vi "BRig_Host_dataRunState__entryAdd_v2.vi"(0 "input_dataPlot":u16[][](array[numeric]), 1 "input_dataTS":u16[][](array[numeric]), 2 "input_idx":i32[](array[numeric]), 4 "input_nTrial":u16, 5 "input_LorR":u16, 7 "input_sSelection":u16, 9 "input_tSelection":u16, 11 "input_tSelectionPlot":u16, 13 "input_iSelection":u16) -> (14 "output_dataPlot":u16[][](array[numeric]), 15 "output_dataTS":u16[][](array[numeric]), 16 "output_idx":i32[](array[numeric]), 18 "output_updatePlot":bool)   [LabVIEW 2014]
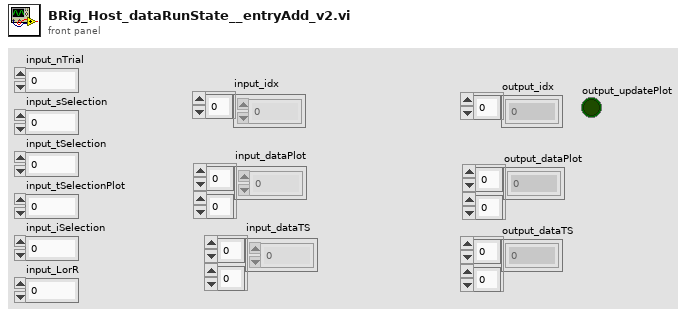
[diagram p1: front panel]
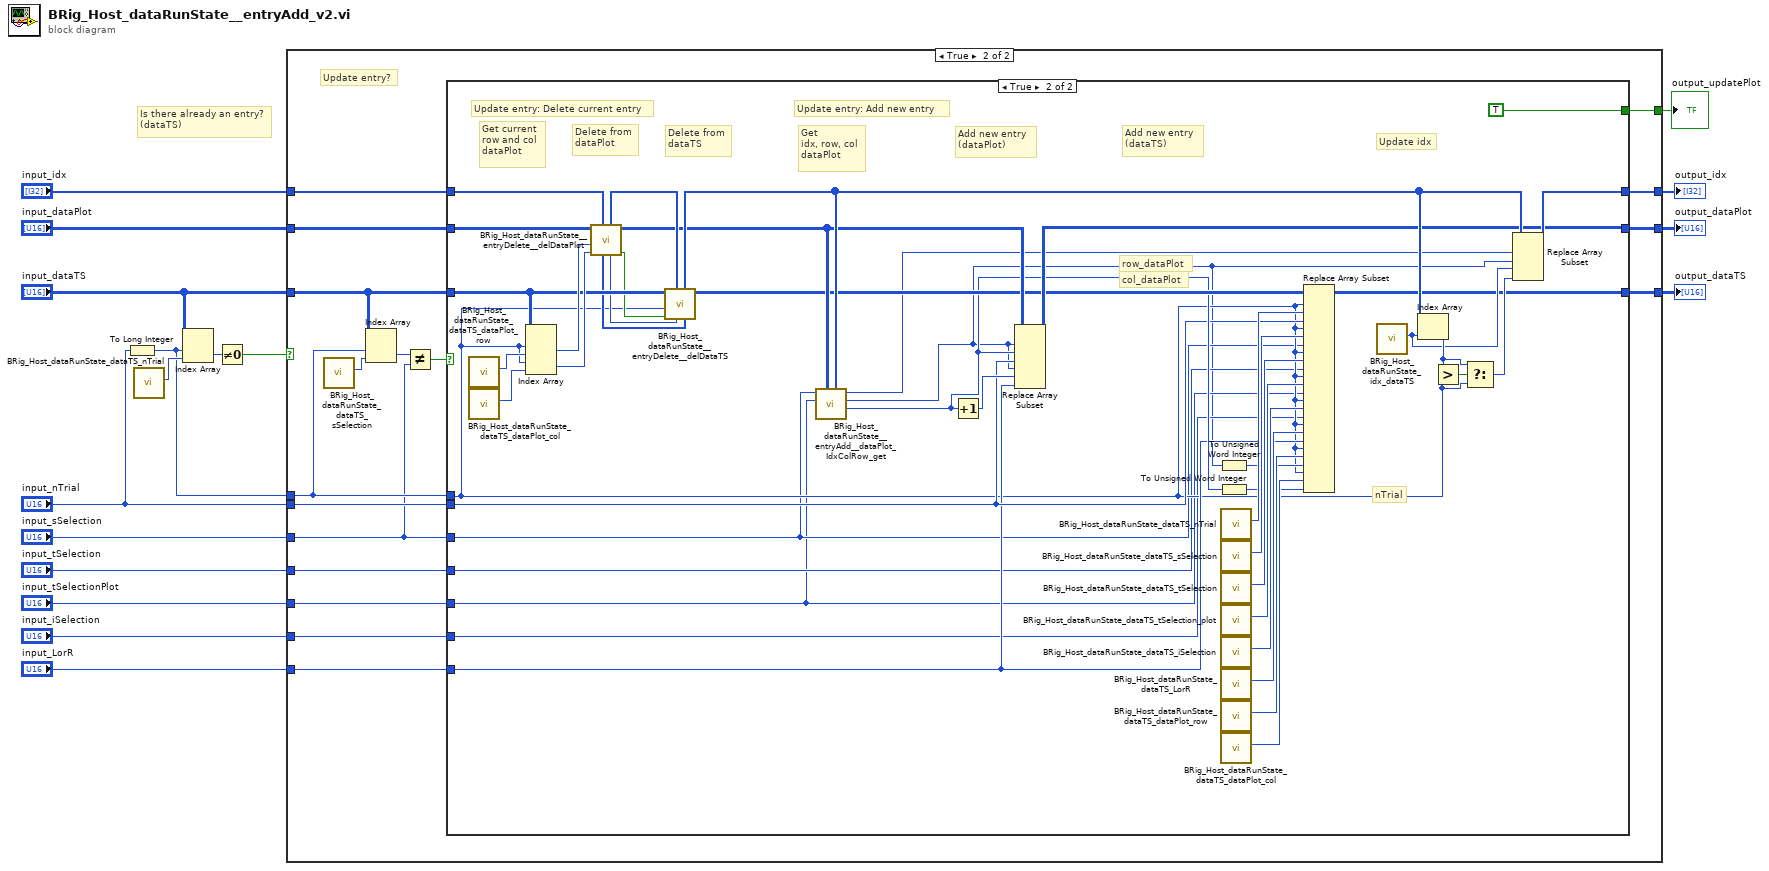
[diagram p0: block diagram]
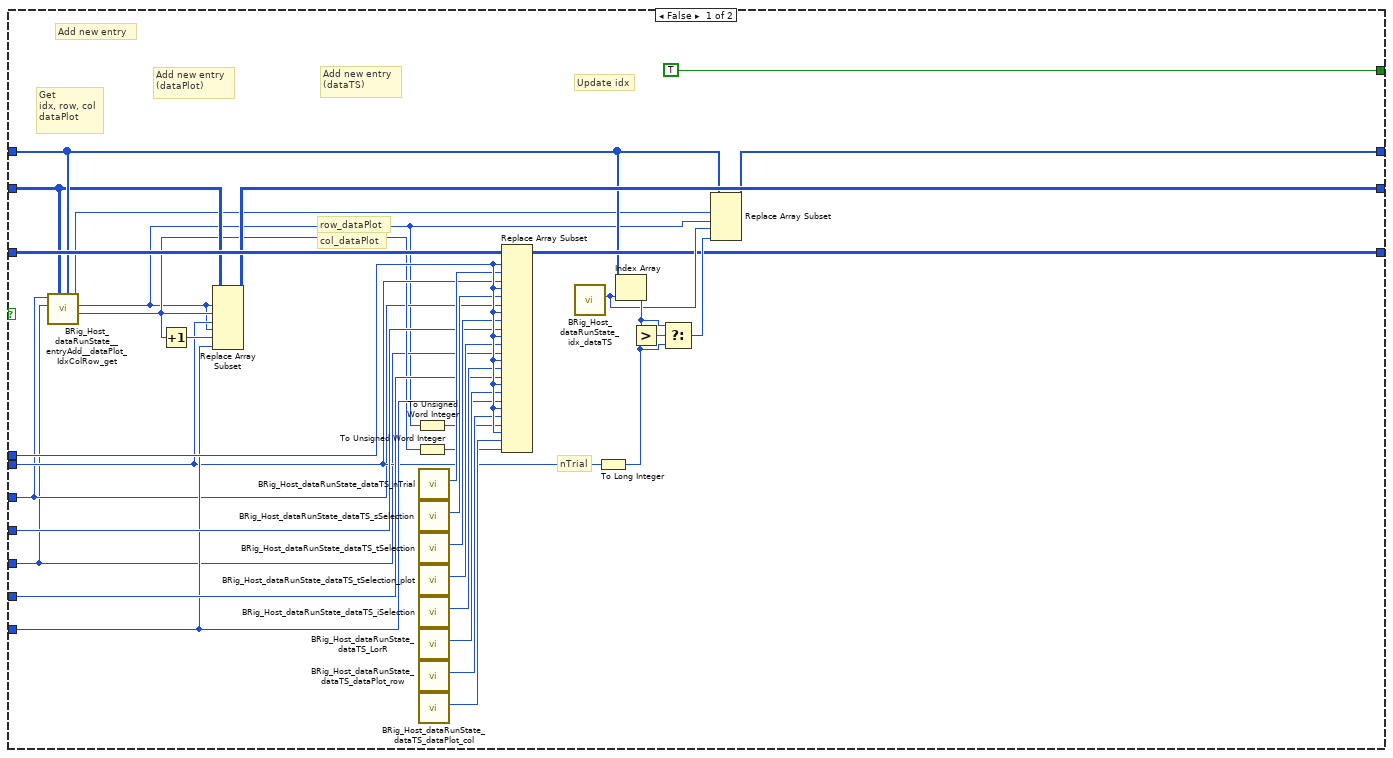
[diagram p2: hidden frame]
diagram:
  # "Is there already an entry?\n(dataTS)"
  n1 = To Long Integer(number="input_nTrial") -> (32bit integer=w13:i32)
  n2 = call "BRig_Host_dataRunState_dataTS_nTrial.vi"() -> ("output_idx_dataTS_nTrial"=w17:i32)  [unwired: 11 in]
  n3 = Index Array(array="input_dataTS", index (row)=w13, index (col)=w17) -> (element=w16:u16)
  n4 = Not Equal To 0?(x=w16) -> (x != 0?=w15:bool)
  n5 = case shown="True" w15 {
    tunnel: "input_nTrial" -> [w27 w57]
    tunnel: w13 -> [w49 w59]
    tunnel: "input_dataTS" -> [w50 w61]
    tunnel: "input_idx" -> [w24 w65]
    tunnel: "input_dataPlot" -> [w23 w63]
    tunnel: "input_sSelection" -> [w20 w51]
    tunnel: "input_tSelectionPlot" -> [w19 w58]
    tunnel: "input_iSelection" -> [w36 w54]
    tunnel: "input_LorR" -> [w35 w56]
    tunnel: [w38 w64] -> w4
    tunnel: [w39 w62] -> w3
    tunnel: [w30 w60] -> w2
    tunnel: "input_tSelection" -> [w37 w55]
    tunnel: [TRUE w53] -> w1
    frame False {
      # "Get\nidx, row, col\ndataPlot"
      # "nTrial"
      # "row_dataPlot"
      # "col_dataPlot"
      # "Update idx"
      # "Add new entry\n(dataPlot)"
      # "Add new entry"
      # "Add new entry\n(dataTS)"
      n6 = call "BRig_Host_dataRunState__entryAdd__dataPlot_IdxColRow_get.vi"("input_idx"=w24, "input_dataPlot"=w23, "input_tSelectionPlot"=w19, "input_sSelection"=w20) -> ("output_col_dataPlot"=w21:i32, "output_row_dataPlot"=w18:i32, "output_idx_dataPlot"=w22:i32)  [unwired: 5 in]
      n7 = Increment(x=w21) -> (x+1=w40:i32)
      n8 = Replace Array Subset(array=w23, new element #1=w27, index (row) #1=w18, index (col) #1=w21, new element #2=w35, index (row) #2=w18, index (col) #2=w40) -> (w39:u16[][])
      n9 = To Unsigned Word Integer(number=w18) -> (unsigned 16bit integer=w29:u16)
      n10 = To Unsigned Word Integer(number=w21) -> (unsigned 16bit integer=w28:u16)
      n11 = call "BRig_Host_dataRunState_dataTS_nTrial.vi"() -> ("output_idx_dataTS_nTrial"=w48:i32)  [unwired: 11 in]
      n12 = call "BRig_Host_dataRunState_dataTS_sSelection.vi"() -> ("output_idx_dataTS_sSelection"=w47:i32)  [unwired: 11 in]
      n13 = call "BRig_Host_dataRunState_dataTS_tSelection.vi"() -> ("output_idx_dataTS_tSelection"=w46:i32)  [unwired: 11 in]
      n14 = call "BRig_Host_dataRunState_dataTS_tSelection_plot.vi"() -> ("output_idx_dataTS_tSelection_plot"=w45:i32)  [unwired: 11 in]
      n15 = call "BRig_Host_dataRunState_dataTS_iSelection.vi"() -> ("output_idx_dataTS_iSelection"=w44:i32)  [unwired: 11 in]
      n16 = call "BRig_Host_dataRunState_dataTS_LorR.vi"() -> ("output_idx_dataTS_LorR"=w43:i32)  [unwired: 11 in]
      n17 = call "BRig_Host_dataRunState_dataTS_dataPlot_row.vi"() -> ("output_idx_dataTS_dataPlot_row"=w42:i32)  [unwired: 11 in]
      n18 = call "BRig_Host_dataRunState_dataTS_dataPlot_col.vi"() -> ("output_idx_dataTS_dataPlot_col"=w41:i32)  [unwired: 11 in]
      n19 = Replace Array Subset(array=w50, new element #1=w27, index (row) #1=w49, index (col) #1=w48, new element #2=w20, index (row) #2=w49, index (col) #2=w47, new element #3=w37, index (row) #3=w49, index (col) #3=w46, new element #4=w19, index (row) #4=w49, index (col) #4=w45, new element #5=w36, index (row) #5=w49, index (col) #5=w44, new element #6=w35, index (row) #6=w49, index (col) #6=w43, new element #7=w29, index (row) #7=w49, index (col) #7=w42, new element #8=w28, index (row) #8=w49, index (col) #8=w41) -> (w30:u16[][])
      n20 = call "BRig_Host_dataRunState_idx_dataTS.vi"() -> ("output_idx_dataTS"=w32:i32)  [unwired: 11 in]
      n21 = To Long Integer(number=w27) -> (32bit integer=w26:i32)
      n22 = Index Array(array=w24, index=w32) -> (element=w33:i32)
      n23 = Greater?(x=w33, y=w26) -> (0:w34:bool)
      n24 = Select(t=w33, s=w34, f=w26) -> (s? t:f=w31:i32)
      n25 = Replace Array Subset(array=w24, new element #1=w18, index #1=w22, new element #2=w31, index #2=w32) -> (w38:i32[])
    }
    frame True {
      # "Update entry?"
      n26 = call "BRig_Host_dataRunState_dataTS_sSelection.vi"() -> ("output_idx_dataTS_sSelection"=w52:i32)  [unwired: 11 in]
      n27 = Index Array(array=w61, index (row)=w59, index (col)=w52) -> (element=w67:u16)
      n28 = Not Equal?(x=w67, y=w51) -> (x != y?=w66:bool)
      n29 = case shown="True" w66 {
        tunnel: w65 -> [w70 w108]
        tunnel: [w70 w86] -> w64
        tunnel: w63 -> [w69 w111]
        tunnel: [w69 w84] -> w62
        tunnel: w61 -> [w68 w107]
        tunnel: [w68 w82] -> w60
        tunnel: w59 -> [_ w77]
        tunnel: w51 -> [_ w76]
        tunnel: w58 -> [_ w74]
        tunnel: w57 -> [_ w79]
        tunnel: w56 -> [_ w78]
        tunnel: w55 -> [_ w75]
        tunnel: w54 -> [_ w73]
        tunnel: [_ TRUE] -> w53
        frame False {
          # "Do nothing"
        }
        frame True {
          # "nTrial"
          # "row_dataPlot"
          # "col_dataPlot"
          # "Update idx"
          # "Add new entry\n(dataPlot)"
          # "Add new entry\n(dataTS)"
          # "Get\nidx, row, col\ndataPlot"
          # "Update entry: Add new entry"
          # "Delete from\ndataTS"
          # "Delete from\ndataPlot"
          # "Get current\nrow and col\ndataPlot"
          # "Update entry: Delete current entry"
          n30 = call "BRig_Host_dataRunState_dataTS_dataPlot_row.vi"() -> ("output_idx_dataTS_dataPlot_row"=w113:i32)  [unwired: 11 in]
          n31 = call "BRig_Host_dataRunState_dataTS_dataPlot_col.vi"() -> ("output_idx_dataTS_dataPlot_col"=w112:i32)  [unwired: 11 in]
          n32 = Index Array(array=w107, index (row) #1=w77, index (col) #1=w113, index (row) #2=w77, index (col) #2=w112) -> (element #1=w109:u16, element #2=w110:u16)
          n33 = call "BRig_Host_dataRunState__entryDelete__delDataPlot.vi"("input_idx"=w108, "input_col_dataPlot"=w110, "input_row_dataPlot"=w109, "input_dataPlot"=w111) -> (0:"output_arrTrials"=w105:bool, "output_dataPlot"=w85:u16[][], "output_arrTrials_length"=w104:i32, "output_idx"=w106:i32[], 6:"output_arrTrials"=w103:i32[])  [unwired: 3 in]
          n34 = call "BRig_Host_dataRunState__entryDelete__delDataTS.vi"(4:"output_arrTrials"=w103, "output_arrTrials_length"=w104, "input_idx"=w106, 8:"output_arrTrials"=w105, "input_nTrial"=w77, "input_dataTS"=w107) -> ("output_dataTS"=w83:u16[][], "output_idx"=w87:i32[])  [unwired: 4 in]
          n35 = call "BRig_Host_dataRunState__entryAdd__dataPlot_IdxColRow_get.vi"("input_idx"=w87, "input_dataPlot"=w85, "input_tSelectionPlot"=w74, "input_sSelection"=w76) -> ("output_col_dataPlot"=w80:i32, "output_row_dataPlot"=w71:i32, "output_idx_dataPlot"=w81:i32)  [unwired: 5 in]
          n36 = Increment(x=w80) -> (x+1=w94:i32)
          n37 = Replace Array Subset(array=w85, new element #1=w79, index (row) #1=w71, index (col) #1=w80, new element #2=w78, index (row) #2=w71, index (col) #2=w94) -> (w84:u16[][])
          n38 = To Unsigned Word Integer(number=w71) -> (unsigned 16bit integer=w89:u16)
          n39 = To Unsigned Word Integer(number=w80) -> (unsigned 16bit integer=w88:u16)
          n40 = call "BRig_Host_dataRunState_dataTS_nTrial.vi"() -> ("output_idx_dataTS_nTrial"=w102:i32)  [unwired: 11 in]
          n41 = call "BRig_Host_dataRunState_dataTS_sSelection.vi"() -> ("output_idx_dataTS_sSelection"=w101:i32)  [unwired: 11 in]
          n42 = call "BRig_Host_dataRunState_dataTS_tSelection.vi"() -> ("output_idx_dataTS_tSelection"=w100:i32)  [unwired: 11 in]
          n43 = call "BRig_Host_dataRunState_dataTS_tSelection_plot.vi"() -> ("output_idx_dataTS_tSelection_plot"=w99:i32)  [unwired: 11 in]
          n44 = call "BRig_Host_dataRunState_dataTS_iSelection.vi"() -> ("output_idx_dataTS_iSelection"=w98:i32)  [unwired: 11 in]
          n45 = call "BRig_Host_dataRunState_dataTS_LorR.vi"() -> ("output_idx_dataTS_LorR"=w97:i32)  [unwired: 11 in]
          n46 = call "BRig_Host_dataRunState_dataTS_dataPlot_row.vi"() -> ("output_idx_dataTS_dataPlot_row"=w96:i32)  [unwired: 11 in]
          n47 = call "BRig_Host_dataRunState_dataTS_dataPlot_col.vi"() -> ("output_idx_dataTS_dataPlot_col"=w95:i32)  [unwired: 11 in]
          n48 = Replace Array Subset(array=w83, new element #1=w79, index (row) #1=w77, index (col) #1=w102, new element #2=w76, index (row) #2=w77, index (col) #2=w101, new element #3=w75, index (row) #3=w77, index (col) #3=w100, new element #4=w74, index (row) #4=w77, index (col) #4=w99, new element #5=w73, index (row) #5=w77, index (col) #5=w98, new element #6=w78, index (row) #6=w77, index (col) #6=w97, new element #7=w89, index (row) #7=w77, index (col) #7=w96, new element #8=w88, index (row) #8=w77, index (col) #8=w95) -> (w82:u16[][])
          n49 = call "BRig_Host_dataRunState_idx_dataTS.vi"() -> ("output_idx_dataTS"=w91:i32)  [unwired: 11 in]
          n50 = Index Array(array=w87, index=w91) -> (element=w92:i32)
          n51 = Greater?(x=w92, y=w77) -> (0:w93:bool)
          n52 = Select(t=w92, s=w93, f=w77) -> (s? t:f=w90:i32)
          n53 = Replace Array Subset(array=w87, new element #1=w71, index #1=w81, new element #2=w90, index #2=w91) -> (w86:i32[])
        }
      }
    }
  }
  "output_idx" <- w4
  "output_dataPlot" <- w3
  "output_dataTS" <- w2
  "output_updatePlot" <- w1
